vi "read_data_from_matfile.vi"(8 "error in":errorcluster, 11 "matFile_info":T1) -> (0 "error out":errorcluster, 1 "content's names":string[](array[string]), 2 "data type":T2[](array[typedef]), 3 "contents":variant[](array[variant]), 4 "number of content":i32, 5 "dimension":i32[][](array[numeric]))   [LabVIEW 2018]
uses:
  MatFile_information.ctl
  type_control.ctl
panel:
  out "Numeric Control":i32
  out "matFile_info 2":T1
  out "data type":i32[](array[numeric])
  out "array name dim":i32[](array[numeric])
  out "dim":i32[](array[numeric])
  out "col":i32[](array[numeric])
  out "row":i32[](array[numeric])
  out "data 3":i8[](array[numeric])
  out "dimension total section":i32[](array[numeric])
  out "type matrix":i32[](array[numeric])
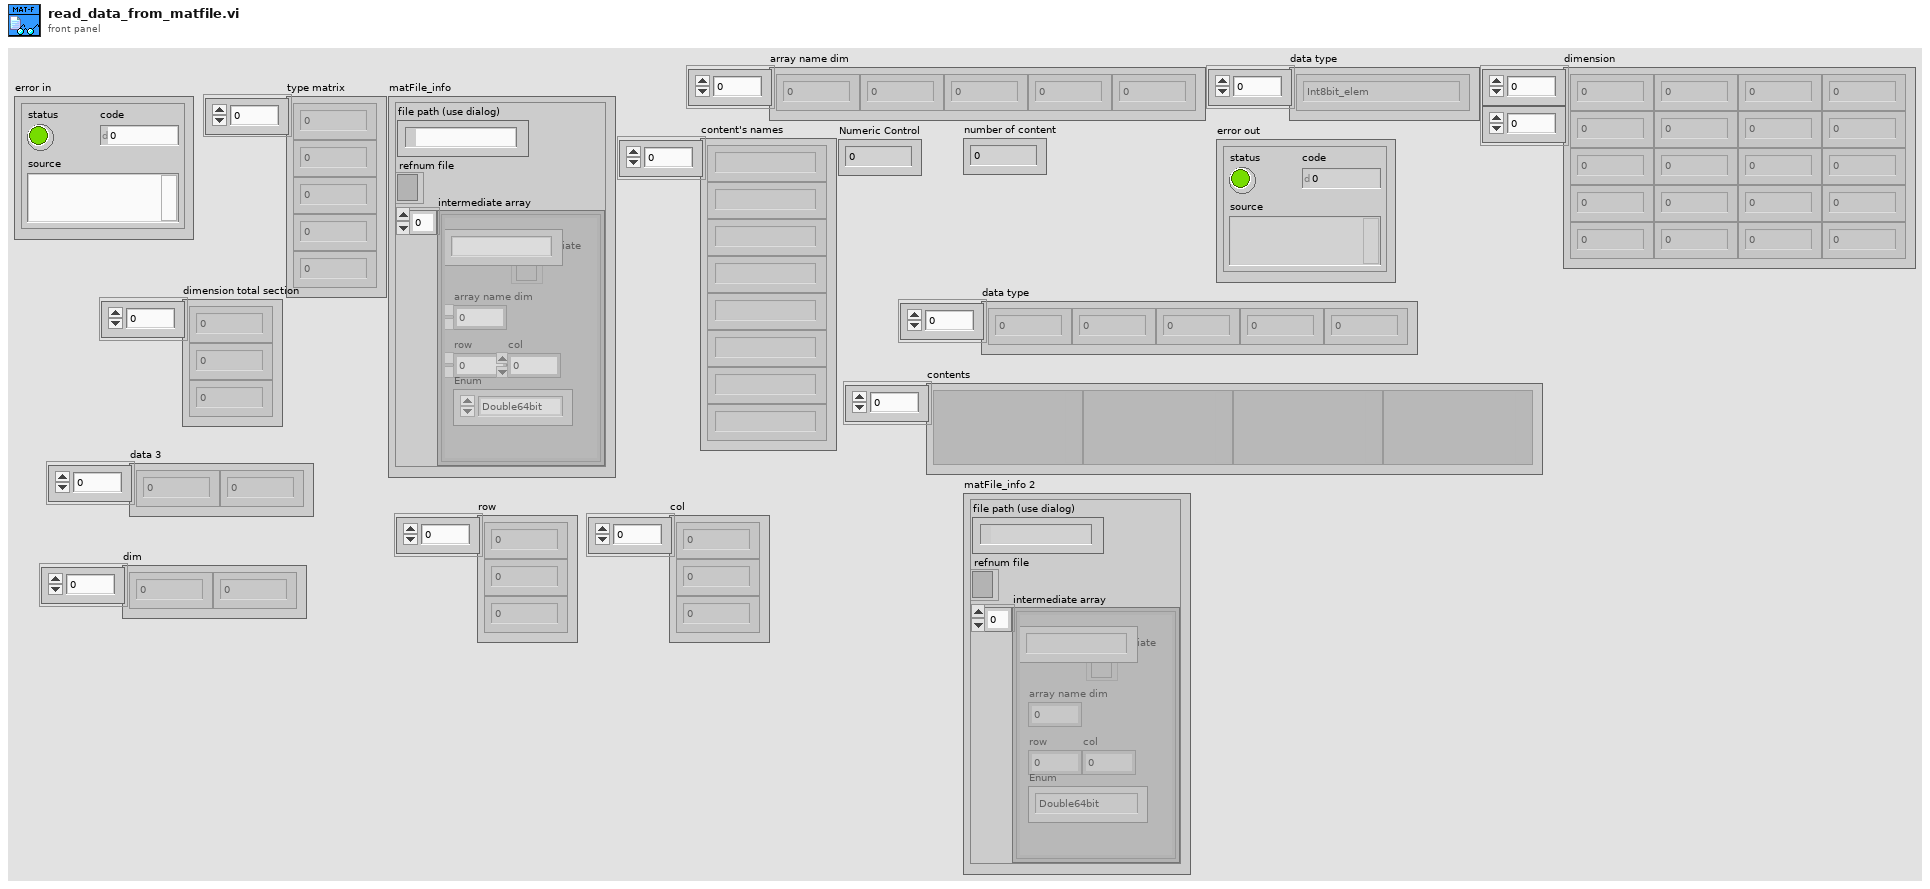
[diagram p1: front panel]
types:
  T1 = typedef "MatFile_information.ctl" = cluster{"file path (use dialog)":path, "refnum file":refnum<file>, "intermediate array":cluster{"intermediate":refnum<file>, "array name dim":i32, "row":i32, "col":i32, "Content":string, "Enum":T2}[]}
  T2 = typedef "type_control.ctl" = enum16{"Int8bit_elem", "Int8bit", "Int64bit_elem", "Int64bit", "Int16bit_elem", "Double64bit_elem", "Int16bit", "Double64bit"}
  T3 = enum16{"big-endian, network order", "native, host order", "little-endian"}
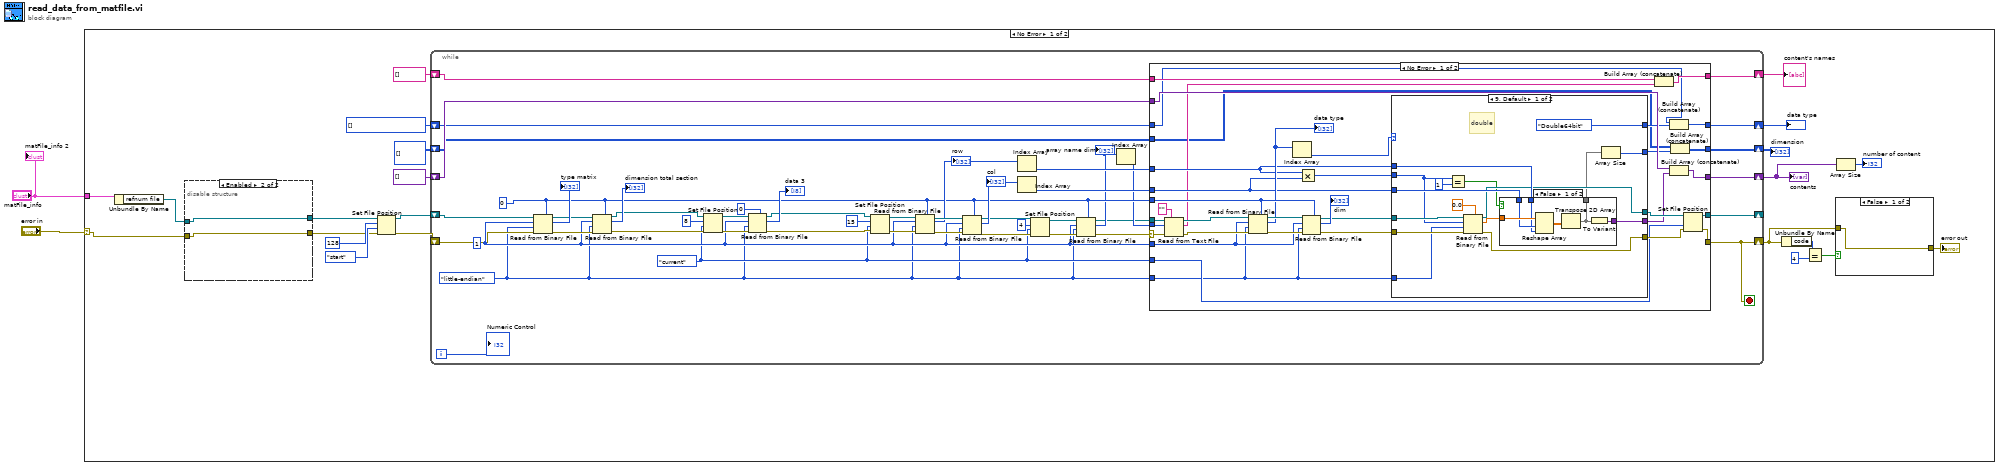
[diagram p0: block diagram]
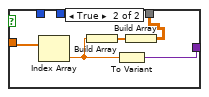
[diagram p2: hidden frame]
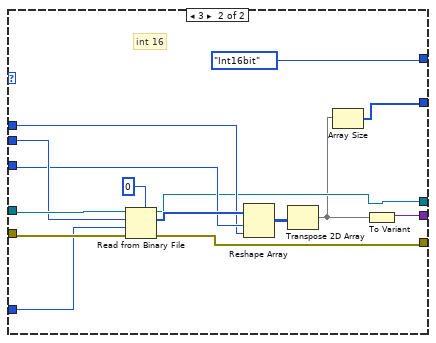
[diagram p3: hidden frame]
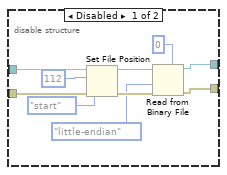
[diagram p5: hidden frame]
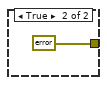
[diagram p6: hidden frame]
diagram:
  n1 = case shown="No Error" "error in" {
    selector: "error in" -> [w10 _]
    tunnel: "matFile_info" -> [w25 _]
    frame No Error {
      w5 = T2[] [] items=["Int8bit_elem", "Int8bit", "Int64bit_elem", "Int64bit", "Int16bit_elem", "Double64bit_elem", "Int16bit", "Double64bit"]
      n2 = Unbundle By Name(w25) -> ("refnum file"=w11:refnum<file>)
      n3 = disable-structure shown="Enabled" {
        disable-tunnel: w11 -> [w167 w169]
        disable-tunnel: w10 -> [w166 w168]
        disable-tunnel: [w164 w168] -> w9
        disable-tunnel: [w162 w169] -> w8
        frame Disabled {
          n4 = Set File Position(offset (in bytes) (0)=i64 112, refnum=w167, from (0:start)=enum16{"start", "end", "current"}."start", error in=w166) -> (refnum out=w163:refnum<file>, error out=w165:errorcluster)
          n5 = Read from Binary File(5:0, 8:w165, 9:T3."little-endian" ("byte order (0:big-endian, network order)"), 11:w163) -> (0:w164:errorcluster, 3:w162:refnum<file>)  [unwired: 2 in, 2 out]
        }
        frame Enabled {
        }
      }
      n6 = Set File Position(offset (in bytes) (0)=i64 128, refnum=w8, from (0:start)=enum16{"start", "end", "current"}."start", error in=w9) -> (refnum out=w12:refnum<file>, error out=w22:errorcluster)
      n7 = while {
        shift-right: [w32] -> w17
        shift-left: w22 -> [w73]
        shift-right: [w34] -> _
        shift-left: w12 -> [w33]
        shift-right: [w31] -> w15
        shift-left: variant[] [] -> [w30]
        shift-right: [w39] -> w13
        shift-left: string[] [] -> [w29]
        shift-right: [w44] -> w18
        shift-left: w5 -> [w28]
        shift-right: [w26] -> w3
        shift-left: i32[][] [] -> [w27]
        i -> [w35]
        stop <- w32 stop-if-true
        w41 = enum16{"start", "end", "current"}."current" ("from (0:start)")
        w47 = 0
        w42 = 1 ("count (1)")
        w40 = T3."little-endian" ("byte order (0:big-endian, network order)")
        n8 = Read from Binary File(5:w47, 8:w73, 9:w40, 10:w42, 11:w33) -> (0:w71:errorcluster, 2:→"type matrix":i32[], 3:w70:refnum<file>)  [unwired: 1 in, 1 out]
        n9 = Read from Binary File(5:w47, 8:w71, 9:w40, 10:w42, 11:w70) -> (0:w66:errorcluster, 2:→"dimension total section":i32[], 3:w67:refnum<file>)  [unwired: 1 in, 1 out]
        n10 = Set File Position(offset (in bytes) (0)=i64 8, refnum=w67, from (0:start)=w41, error in=w66) -> (refnum out=w64:refnum<file>, error out=w65:errorcluster)
        n11 = Read from Binary File(5:i8 0, 8:w65, 9:w40, 10:w42, 11:w64) -> (0:w57:errorcluster, 2:→"data 3":i8[], 3:w58:refnum<file>)  [unwired: 1 in, 1 out]
        n12 = Set File Position(offset (in bytes) (0)=i64 15, refnum=w58, from (0:start)=w41, error in=w57) -> (refnum out=w61:refnum<file>, error out=w60:errorcluster)
        n13 = Read from Binary File(5:w47, 8:w60, 9:w40, 10:w42, 11:w61) -> (0:w55:errorcluster, 2:w54:i32[], 3:w56:refnum<file>)  [unwired: 1 in, 1 out]
        "row" <- w54
        n14 = Read from Binary File(5:w47, 8:w55, 9:w40, 10:w42, 11:w56) -> (0:w51:errorcluster, 2:w53:i32[], 3:w52:refnum<file>)  [unwired: 1 in, 1 out]
        "col" <- w53
        n15 = Index Array(array=w54) -> (element=w46:i32)  [unwired: 1 in]
        n16 = Index Array(array=w53) -> (element=w45:i32)  [unwired: 1 in]
        n17 = Set File Position(offset (in bytes) (0)=i64 4, refnum=w52, from (0:start)=w41, error in=w51) -> (refnum out=w48:refnum<file>, error out=w49:errorcluster)
        n18 = Read from Binary File(5:w47, 8:w49, 9:w40, 10:w42, 11:w48) -> (0:w43:errorcluster, 2:w38:i32[], 3:w36:refnum<file>)  [unwired: 1 in, 1 out]
        "array name dim" <- w38
        n19 = Index Array(array=w38) -> (element=w37:i32)  [unwired: 1 in]
        n20 = case shown="No Error" w43 {
          selector: w43 -> [w96 w157]
          tunnel: w47 -> [w105 _]
          tunnel: w46 -> [w100 _]
          tunnel: w45 -> [w99 _]
          tunnel: [w79 w154] -> w44
          tunnel: w42 -> [w93 _]
          tunnel: w41 -> [w92 _]
          tunnel: w40 -> [w91 _]
          tunnel: [w81 w153] -> w39
          tunnel: w37 -> [w89 _]
          tunnel: w36 -> [w88 w156]
          tunnel: [w87 w156] -> w34
          tunnel: [w86 w157] -> w32
          tunnel: [w84 w155] -> w31
          tunnel: w30 -> [w83 w155]
          tunnel: w29 -> [w78 w153]
          tunnel: w28 -> [w77 w154]
          tunnel: [w75 w152] -> w26
          tunnel: w27 -> [w74 w152]
          frame No Error {
            n21 = Read from Text File(prompt (Open existing file)="", file (use dialog)=w88, count=w89, error in=w96) -> (refnum out=w94:refnum<file>, text=w82:string, error out=w95:errorcluster)  [unwired: 1 out]
            n22 = Read from Binary File(5:w105, 8:w95, 9:w91, 10:w93, 11:w94) -> (0:w103:errorcluster, 2:w102:i32[], 3:w104:refnum<file>)  [unwired: 1 in, 1 out]
            "data type" <- w102
            n23 = Index Array(array=w102) -> (element=w101:i32)  [unwired: 1 in]
            n24 = Multiply(x=w100, y=w99) -> (x*y=w106:i32)
            n25 = Read from Binary File(5:w105, 8:w103, 9:w91, 10:w93, 11:w104) -> (0:w107:errorcluster, 2:→"dim":i32[], 3:w108:refnum<file>)  [unwired: 1 in, 1 out]
            n26 = case shown="9, Default" w101 {
              tunnel: w108 -> [w125 w148]
              tunnel: w107 -> [w124 w147]
              tunnel: w106 -> [w114 w145]
              tunnel: w91 -> [w123 w146]
              tunnel: [type_control."Double64bit" ("Enum") type_control."Int16bit" ("Enum")] -> w80
              tunnel: w100 -> [w119 w143]
              tunnel: w99 -> [w120 w144]
              tunnel: [w118 w141] -> w85
              tunnel: [w117 w140] -> w98
              tunnel: [w116 w142] -> w97
              tunnel: [w110 w137] -> w76
              frame 9, Default {
                # "double"
                n27 = Equal?(x=w114, y=1) -> (x = y?=w112:bool)
                n28 = Read from Binary File(5:0.0, 8:w124, 9:w123, 10:w114, 11:w125) -> (0:w117:errorcluster, 2:w121:dbl[], 3:w116:refnum<file>)  [unwired: 1 in, 1 out]
                n29 = case shown="False" w112 {
                  tunnel: w121 -> [w130 w136]
                  tunnel: w120 -> [w129 _]
                  tunnel: w119 -> [w128 _]
                  tunnel: [w127 w135] -> w118
                  tunnel: [w126 w132] -> w111
                  frame False {
                    n30 = Reshape Array(w130, w129, w128) -> (w131:dbl[][])
                    n31 = Transpose 2D Array(2D array=w131) -> (transposed array=w126:dbl[][])
                    n32 = To Variant(anything=w126) -> (Variant=w127:variant)
                  }
                  frame True {
                    n33 = Index Array(array=w136) -> (element=w134:dbl)  [unwired: 1 in]
                    n34 = Build Array(w134) -> (w133:dbl[])
                    n35 = To Variant(anything=w134) -> (Variant=w135:variant)
                    n36 = Build Array(w133) -> (w132:dbl[][])
                  }
                }
                n37 = Array Size(array=w111) -> (size(s)=w110:i32[])
              }
              frame 3 {
                # "int 16"
                n38 = Read from Binary File(5:i16 0, 8:w147, 9:w146, 10:w145, 11:w148) -> (0:w140:errorcluster, 2:w149:i16[], 3:w142:refnum<file>)  [unwired: 1 in, 1 out]
                n39 = Reshape Array(w149, w144, w143) -> (w150:i16[][])
                n40 = Transpose 2D Array(2D array=w150) -> (transposed array=w138:i16[][])
                n41 = Array Size(array=w138) -> (size(s)=w137:i32[])
                n42 = To Variant(anything=w138) -> (Variant=w141:variant)
              }
            }
            n43 = Build Array (concatenate)(w78, w82) -> (w81:string[])
            n44 = Build Array (concatenate)(w77, w80) -> (w79:T2[])
            n45 = Build Array (concatenate)(w83, w85) -> (w84:variant[])
            n46 = Build Array (concatenate)(w74, w76) -> (w75:i32[][])
            n47 = Set File Position(refnum=w97, from (0:start)=w92, error in=w98) -> (refnum out=w87:refnum<file>, error out=w86:errorcluster)  [unwired: 1 in]
          }
          frame Error {
          }
        }
        "Numeric Control" <- w35
      }
      "contents" <- w15
      "data type" <- w18
      "content's names" <- w13
      "dimension" <- w3
      n48 = Unbundle By Name(w17) -> ("code"=w21:i32)
      n49 = Equal?(x=w21, y=4) -> (x = y?=w19:bool)
      n50 = case shown="False" w19 {
        tunnel: [w170 errorcluster {"status"=FALSE, "code"=0, "source"=""} ("error constant")] -> w16
        tunnel: w17 -> [w170 _]
        frame False {
        }
        frame True {
        }
      }
      "error out" <- w16
      n51 = Array Size(array=w15) -> (size(s)=→"number of content":i32)
    }
    frame Error {
    }
  }
  "matFile_info 2" <- "matFile_info"
